vi "XTicks.vi"(4 "Properties":T1={"Text"={"Color"=2147483647, "Background Color"=2147483647, "Font Size (points)"=0, "Font Style"=enum."Automatic", "Rotation Angle"=nan}} {"Text"."Background Color" items=["Automatic"=2147483647, "Black"=0, "White"=16777215, "Red"=16711680, "Green"=2263842, "Blue"=255, "Cyan"=65535, "Magenta"=16711935, "Yellow"=16776960]; "Text"."Font Size (points)" items=["Automatic"=0, "XX-Small"=-1, "X-Small"=-2, "Small"=-3, "Medium"=-4, "Large"=-5, "X-Large"=-6, "XX-Large"=-7]; "Text"."Color" items=["Automatic"=2147483647, "Black"=0, "White"=16777215, "Red"=16711680, "Green"=2263842, "Blue"=255, "Cyan"=65535, "Magenta"=16711935, "Yellow"=16776960]}, 8 "error in (no error)":errorcluster, 9 "Tick Labels":string[](array[string]), 10 "Tick Locations":dbl[](array[numeric]), 11 "Plot ID":T6 format="%x") -> (0 "error out":errorcluster, 3 "Plot ID Out":T6 format="%x")   [LabVIEW 2013, in "Advanced Plotting Toolkit.lvlib"]
doc: "Set the location of the X axis tick marks, and optionally their labels."
uses:
  Advanced Plotting Toolkit.lvlib
  typedefs/PlotID.ctl
  TicksProperties.ctl
  properties/Text.ctl
  typedefs/PlotColor.ctl
  properties/Text_FontSize.ctl
  properties/Text_FontStyle.ctl
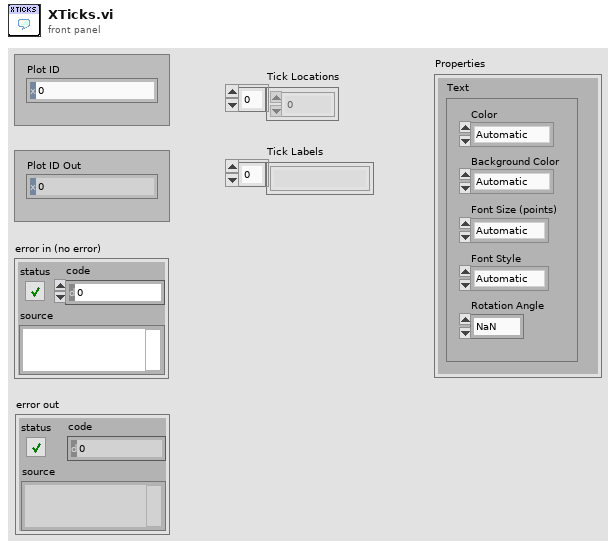
[diagram p1: front panel]
types:
  T1 = typedef "Advanced Plotting Toolkit.lvlib/TicksProperties.ctl" = cluster{"Text":T2}
  T2 = typedef "Advanced Plotting Toolkit.lvlib/Text.ctl" = cluster{"Color":T3, "Background Color":T3, "Font Size (points)":T4, "Font Style":T5, "Rotation Angle":dbl}
  T3 = typedef "Advanced Plotting Toolkit.lvlib/PlotColor.ctl" = u32
  T4 = typedef "Advanced Plotting Toolkit.lvlib/Text_FontSize.ctl" = i32
  T5 = typedef "Advanced Plotting Toolkit.lvlib/Text_FontStyle.ctl" = enum16{"Automatic", "Normal", "Italic", "Bold"}
  T6 = typedef "Advanced Plotting Toolkit.lvlib/PlotID.ctl" = i32
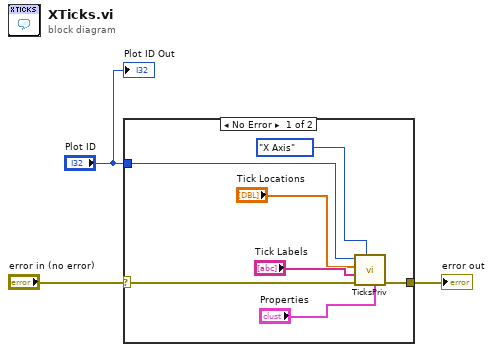
[diagram p0: block diagram]
diagram:
  n1 = case shown="No Error" "error in (no error)" {
    selector: "error in (no error)" -> [w10 w11]
    tunnel: "Plot ID" -> [w5 _]
    tunnel: [w9 w11] -> w1
    frame No Error {
      n2 = call "TicksPriv.vi"("Tick Properties"="Properties", "Axis"=enum16{"X Axis", "Y Axis"}."X Axis", "error in (no error)"=w10, "Tick Labels"="Tick Labels", "Tick Locations"="Tick Locations", "Plot ID"=w5) -> ("error out"=w9:errorcluster)  [unwired: 5 in]
    }
    frame Error {
    }
  }
  "error out" <- w1
  "Plot ID Out" <- "Plot ID"
